vi "nanocal-frontend-tcplink-server-LV18.vi.vi"() -> ()   [LabVIEW 2018]
doc: "Demonstrates how to set up a basic TCP connection, send data to the specified port once a connection has been established, and terminate the connection once the data has been sent. This VI is designed to stop if the TCP connection is terminated. The data sent in this example is an array of random numbers."
uses:
  nanocal server folder LV18/icicle.ctl
  nanocal server folder LV18/publisher action.ctl
panel:
  in  "Tab Control":enum32{"Page 1", "Page 2"}(tab)
  in  "Stop":bool
  in  "port":u16=6340
  in  "timeout (ms)":i32=30000
  in  "wait (ms)":u32=100
  out "nanocal data array OUT":T1[](array[typedef])
  # "nanocal tcplink -- Server"
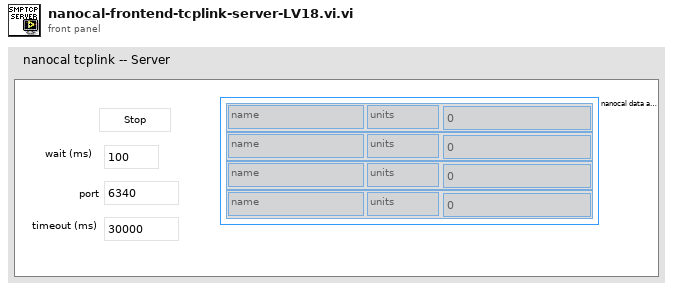
[diagram p1: front panel]
types:
  T1 = typedef "icicle.ctl" = cluster{"name":string, "units":string, "data":dbl}
  T2 = typedef "publisher action.ctl" = enum16{"set", "get", "init", "check"}
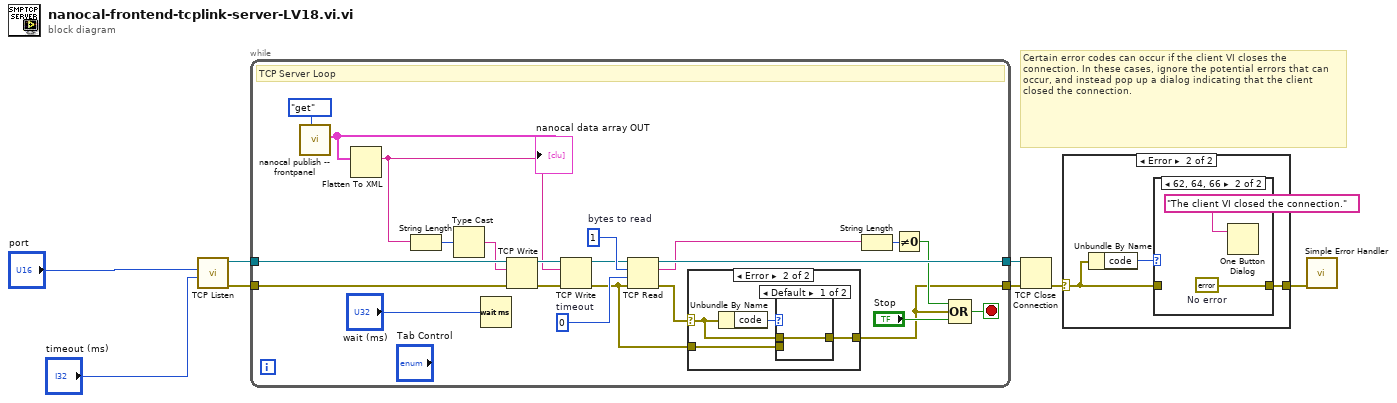
[diagram p0: block diagram]
diagram:
  # "Certain error codes can occur if the client VI closes the connection. In these cases, ignore the potential errors that can occur, and instead pop up a dialog indicating that the client closed the connection."
  n1 = call <vilib>:"TCP Listen.vi"("timeout ms (wait forever: -1)"="timeout (ms)", "port"="port") -> ("error out"=w3:errorcluster, "connection ID"=w4:refnum<k5>)  [unwired: 5 in, 3 out]
  n2 = while {
    tunnel: [w13] -> w7
    tunnel: [w19] -> w8
    tunnel: w4 -> [w30]
    tunnel: w3 -> [w23]
    stop <- w24 stop-if-true
    w18 = 0  # timeout
    w21 = 1  # bytes to read
    # "TCP Server Loop"
    n3 = call "nanocal publish -- frontpanel.vi"("publisher action"=publisher_action."get") -> ("nanocal data array OUT"=w10:T1[])  [unwired: 10 in]
    "nanocal data array OUT" <- w10
    n4 = Flatten To XML(anything=w10) -> (xml string=w9:string)
    n5 = String Length(string=w9) -> (length=w27:i32)
    n6 = Type Cast(x=w27) -> (*(type *) &x=w26:string)  [unwired: 1 out]
    n7 = Wait (ms)(milliseconds to wait="wait (ms)") -> ()  [unwired: 1 out]
    n8 = TCP Write(connection ID=w30, data in=w26, error in (no error)=w23) -> (connection ID out=w29:refnum<k5>, error out=w28:errorcluster)  [unwired: 2 out]
    n9 = TCP Write(connection ID=w29, data in=w9, error in (no error)=w28) -> (connection ID out=w20:refnum<k5>, error out=w12:errorcluster)  [unwired: 2 out]
    n10 = TCP Read(connection ID=w20, bytes to read=w21, error in (no error)=w12, 9:w18) -> (connection ID out=w19:refnum<k5>, data out=w16:string, error out=w14:errorcluster)  [unwired: 1 out]
    n11 = case shown="Error" w14 {
      selector: w14 -> [w31 w34]
      tunnel: [w31 w32] -> w13
      tunnel: w12 -> [_ w33]
      frame No Error {
      }
      frame Error {
        n12 = Unbundle By Name(w34) -> ("code"=w35:i32)
        n13 = case shown="Default" w35 {
          tunnel: w34 -> [w36 _]
          tunnel: w33 -> [_ w37]
          tunnel: [w36 w37] -> w32
          frame Default {
          }
          frame 56 {
          }
        }
      }
    }
    n14 = String Length(string=w16) -> (length=w17:i32)
    n15 = Not Equal To 0?(x=w17) -> (x != 0?=w15:bool)
    n16 = Compound Arithmetic op=OR(w15, w13, "Stop") -> (w24:bool)
  }
  n17 = TCP Close Connection(connection ID=w8, error in (no error)=w7) -> (error out=w6:errorcluster)  [unwired: 2 out]
  n18 = case shown="Error" w6 {
    selector: w6 -> [w38 w40]
    tunnel: [w38 w39] -> w5
    frame No Error {
    }
    frame Error {
      n19 = Unbundle By Name(w40) -> ("code"=w41:i32)
      n20 = case shown="62, 64, 66" w41 {
        tunnel: w40 -> [w42 _]
        tunnel: [w42 w44] -> w39
        frame Default {
        }
        frame 62, 64, 66 {
          w44 = errorcluster {"status"=FALSE, "code"=0, "source"=""}  # No error
          n21 = One Button Dialog(message="The client VI closed the connection." ("Client Closed")) -> ()  [unwired: 1 in, 1 out]
        }
      }
    }
  }
  n22 = call <vilib>:"Simple Error Handler.vi"("error in (no error)"=w5) -> ()  [unwired: 1 in, 8 out]
